vi "Do.vi"(8 "error in (no error)":errorcluster, 10 "Actor in":refnum<class "Actor.lvclass">, 11 "Unregister Variant Msg":refnum<class "Unregister Sensor Number Msg.lvclass">) -> (0 "error out":errorcluster, 2 "Actor out":refnum<class "Actor.lvclass">)   [LabVIEW 2013, in "Main Model.lvlib" / "Unregister Sensor Number Msg.lvclass"]
doc: "(<B>Filename</B>: Actor Framework.lvlib:Message.lvclass:Do.vi)\n\nDefines what a message does when it is received by an actor. Generally, a message instructs an actor to invoke one of its methods.\n\nBy default, this method does nothing. A child class must override it to define behavior. Create a child class by using the Actor Framework Message Maker dialog box."
uses:
  Unregister Sensor Number Msg.lvclass
  <vilib>/ActorFramework/Actor/Actor.lvclass
  Main Model/Main Model.lvclass
  <vilib>/ActorFrameworkMVC/View Observer/Unregistration Message/Unregistration Message.lvclass/Unregistration Message.ctl
  <vilib>/ActorFramework/Message Enqueuer/Message Enqueuer.lvclass
  <vilib>/ActorFrameworkMVC/View Observer/Unregistration Message/Unregistration Message.lvclass
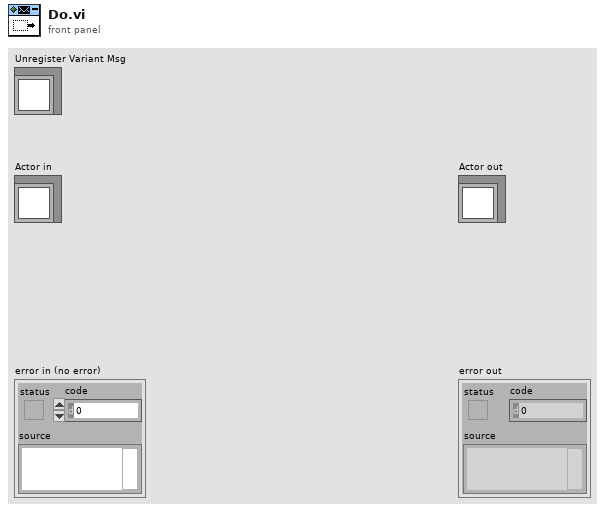
[diagram p1: front panel]
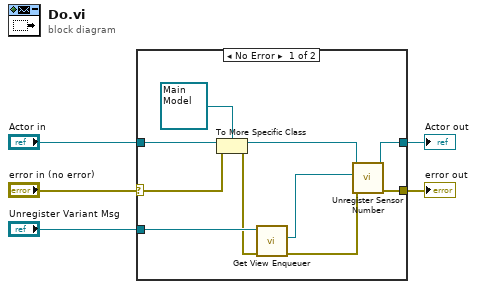
[diagram p0: block diagram]
diagram:
  n1 = case shown="No Error" "error in (no error)" {
    selector: "error in (no error)" -> [w8 w17]
    tunnel: "Unregister Variant Msg" -> [w15 _]
    tunnel: "Actor in" -> [w14 w16]
    tunnel: [w11 w16] -> w1
    tunnel: [w9 w17] -> w2
    frame No Error {
      n2 = To More Specific Class(target class=refnum<class "Main Model.lvclass"> refnum ("Model Actor.lvlib:Model Actor.lvclass"), reference=w14, error in=w8) -> (specific class reference=w12:refnum<class "Main Model.lvclass">, error out=w7:errorcluster)
      n3 = call <vilib>:"Get View Enqueuer.vi"("error in (no error)"=w7, "Unregistration Message in"=w15) -> ("error out"=w6:errorcluster, "View Enqueuer"=w10:refnum<class "Message Enqueuer.lvclass">)  [unwired: 7 in, 1 out]
      n4 = call "Unregister Sensor Number.vi"("error in (no error)"=w6, "View Enqueuer"=w10, "Main Model in"=w12) -> ("error out"=w9:errorcluster, "Main Model out"=w11:refnum<class "Main Model.lvclass">)  [unwired: 7 in]
    }
    frame Error {
    }
  }
  "error out" <- w2
  "Actor out" <- w1
